vi "WriteCounters.vi"(1 "Counters":T2(array[cluster]), 2 "refnum":T1) -> (0 "refnum out":T1)   [LabVIEW 2018]
uses:
  <vilib>/Utility/config.llb/NI_LVConfig.lvlib
  <vilib>/Utility/config.llb/Write Key (String).vi
  <vilib>/Utility/config.llb/Config Data RefNum.ctl
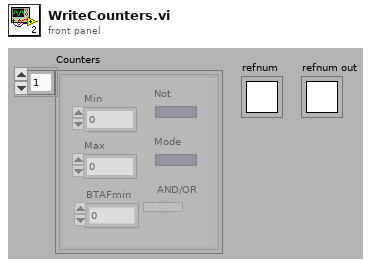
[diagram p1: front panel]
types:
  T1 = typedef "NI_LVConfig.lvlib/Config Data RefNum.ctl" = refnum<k1>
  T2 = cluster{"Min":i16, "Max":i16, "Not":bool, "Mode":bool, "BTAFmin":i16, "AND/OR":bool}[]
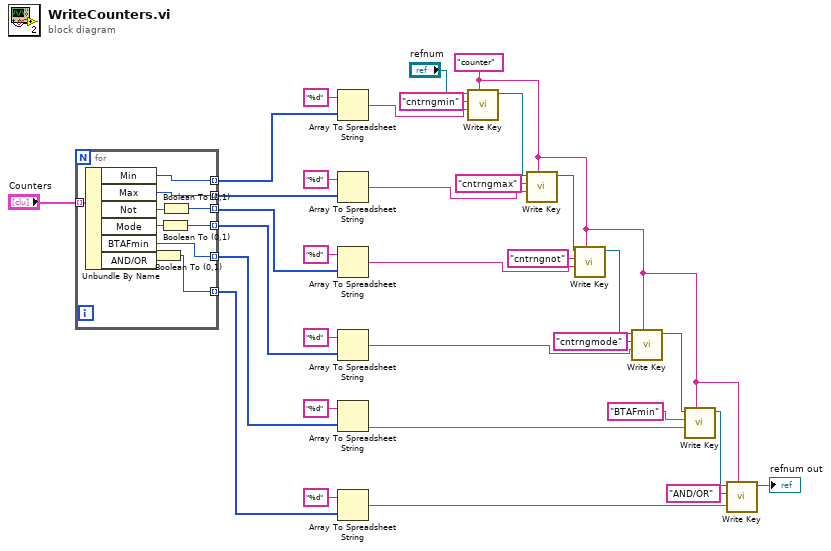
[diagram p0: block diagram]
diagram:
  w5 = "counter" ("section")
  n1 = for {
    tunnel: "Counters" -> [w43] mode=indexing
    tunnel: [w42] -> w32 mode=indexing
    tunnel: [w41] -> w31 mode=indexing
    tunnel: [w38] -> w30 mode=indexing
    tunnel: [w37] -> w29 mode=indexing
    tunnel: [w36] -> w11 mode=indexing
    tunnel: [w34] -> w7 mode=indexing
    n2 = Unbundle By Name(w43) -> ("Min"=w42:i16, "Max"=w41:i16, "Not"=w40:bool, "Mode"=w39:bool, "BTAFmin"=w36:i16, "AND/OR"=w35:bool)
    n3 = Boolean To (0,1)(Boolean=w35) -> (0, 1=w34:i16)
    n4 = Boolean To (0,1)(Boolean=w39) -> (0, 1=w37:i16)
    n5 = Boolean To (0,1)(Boolean=w40) -> (0, 1=w38:i16)
  }
  n6 = Array To Spreadsheet String(array=w32, 3:"%d" ("format string")) -> (spreadsheet string=w16:string)  [unwired: 1 in]
  n7 = Array To Spreadsheet String(array=w31, 3:"%d" ("format string")) -> (spreadsheet string=w15:string)  [unwired: 1 in]
  n8 = Array To Spreadsheet String(array=w30, 3:"%d" ("format string")) -> (spreadsheet string=w14:string)  [unwired: 1 in]
  n9 = Array To Spreadsheet String(array=w29, 3:"%d" ("format string")) -> (spreadsheet string=w13:string)  [unwired: 1 in]
  n10 = Array To Spreadsheet String(array=w11, 3:"%d" ("format string")) -> (spreadsheet string=w9:string)  [unwired: 1 in]
  n11 = Array To Spreadsheet String(array=w7, 3:"%d" ("format string")) -> (spreadsheet string=w3:string)  [unwired: 1 in]
  n12 = call-poly <vilib>:"Write Key.vi"("section"=w5, "value"=w16, "key"="cntrngmin", "refnum"="refnum") -> ("refnum out"=w23:T1)  [unwired: 5 in, 2 out]
  n13 = call-poly <vilib>:"Write Key.vi"("section"=w5, "value"=w15, "key"="cntrngmax", "refnum"=w23) -> ("refnum out"=w22:T1)  [unwired: 5 in, 2 out]
  n14 = call-poly <vilib>:"Write Key.vi"("section"=w5, "value"=w14, "key"="cntrngnot", "refnum"=w22) -> ("refnum out"=w21:T1)  [unwired: 5 in, 2 out]
  n15 = call-poly <vilib>:"Write Key.vi"("section"=w5, "value"=w13, "key"="cntrngmode", "refnum"=w21) -> ("refnum out"=w10:T1)  [unwired: 5 in, 2 out]
  n16 = call-poly <vilib>:"Write Key.vi"("section"=w5, "value"=w9, "key"="BTAFmin", "refnum"=w10) -> ("refnum out"=w1:T1)  [unwired: 5 in, 2 out]
  n17 = call-poly <vilib>:"Write Key.vi"("section"=w5, "value"=w3, "key"="AND/OR", "refnum"=w1) -> ("refnum out"=→"refnum out":T1)  [unwired: 5 in, 2 out]
